vi "relase.vi"(11 "hDevice":i32) -> ()   [LabVIEW 2012]
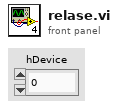
[diagram p1: front panel]
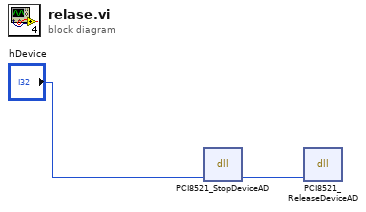
[diagram p0: block diagram]
diagram:
  n1 = dll-call lib="PCI8521_32" fn="PCI8521_StopDeviceAD" label="StopDeviceAD"("hDevice"="hDevice") -> ("hDevice"=w1:i32)  [unwired: 4 in, 2 out]
  n2 = dll-call lib="PCI8521_32" fn="PCI8521_ReleaseDeviceAD" label="ReleaseDeviceAD"("hDevice"=w1) -> ()  [unwired: 5 in, 2 out]
